vi "Initialise Service.vi"(11 "Service Action Base in":refnum<class "Service Action Base.lvclass">) -> (3 "Service Action Base out":refnum<class "Service Action Base.lvclass">)   [LabVIEW 2016, in "Assert API Components.lvlib" / "Assert Service.lvlib" / "Service Action Base.lvclass"]
uses:
  Service Action Base.lvclass
  Service Action Base.lvclass/Service Action Base.ctl
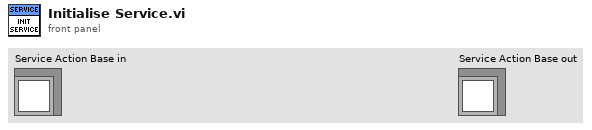
[diagram p1: front panel]
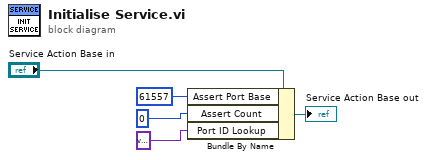
[diagram p0: block diagram]
diagram:
  n1 = Bundle By Name(cluster="Service Action Base in", "Assert Port Base"=u16 61557, "Assert Count"=u16 0, "Port ID Lookup"=variant) -> (→"Service Action Base out":refnum<class "Service Action Base.lvclass">)
